vi "Psych Chart Look-up BY RH.vi"(0 "Relative Humidity [%]":dbl=72.0, 5 "Air Pressure [psia]":dbl=14.7, 7 "1st known value":dbl=55.0, 12 "1st Known Index":u16(ring) items=["DB", "WB", "RH", "HR", "Gr", "Vol", "h", "Dp"]) -> (8 "Output Array":dbl[](array[numeric]))   [LabVIEW 2020]
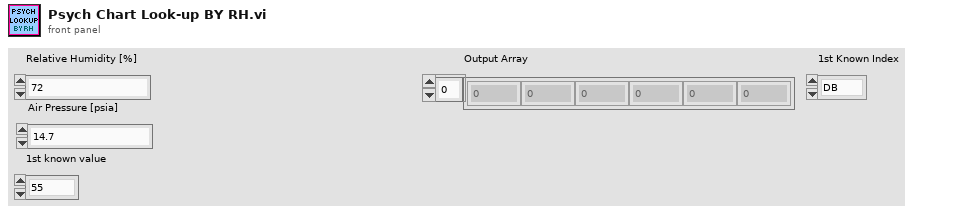
[diagram p1: front panel]
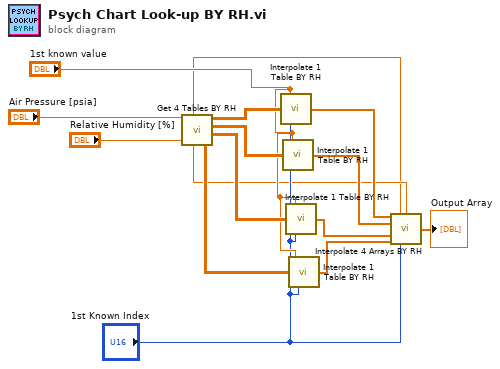
[diagram p0: block diagram]
diagram:
  n1 = call "Get 4 Tables BY RH.vi"("Air Pressure [psia]"="Air Pressure [psia]", "Relative Humidity [%]"="Relative Humidity [%]") -> ("Pressure Z"=w2:dbl, "RH Z"=w3:dbl, "HP Higher RH Psych Table"=w13:dbl[][], "HP Lower RH Psych Table"=w12:dbl[][], "LP Higher RH Psych Table"=w11:dbl[][], "LP Lower RH Psych Table"=w10:dbl[][])  [unwired: 1 in]
  n2 = call "Interpolate 1 Table BY RH.vi"("First Known Value"="1st known value", "Psych Table, 1 Press., 1 RH"=w13, "First Known Index"="1st Known Index") -> ("Output Array"=w9:dbl[])  [unwired: 12 in]
  n3 = call "Interpolate 1 Table BY RH.vi"("First Known Value"="1st known value", "Psych Table, 1 Press., 1 RH"=w12, "First Known Index"="1st Known Index") -> ("Output Array"=w8:dbl[])  [unwired: 12 in]
  n4 = call "Interpolate 1 Table BY RH.vi"("First Known Value"="1st known value", "Psych Table, 1 Press., 1 RH"=w11, "First Known Index"="1st Known Index") -> ("Output Array"=w7:dbl[])  [unwired: 12 in]
  n5 = call "Interpolate 1 Table BY RH.vi"("First Known Value"="1st known value", "Psych Table, 1 Press., 1 RH"=w10, "First Known Index"="1st Known Index") -> ("Output Array"=w6:dbl[])  [unwired: 12 in]
  n6 = call "Interpolate 4 Arrays BY RH.vi"("HP Higher RH Array"=w9, "Pressure Z"=w2, "RH Z"=w3, "HP Lower RH Array"=w8, "LP Higher RH Array"=w7, "LP Lower RH Array"=w6, "1st Known Index"="1st Known Index") -> ("Output Array"=→"Output Array":dbl[])  [unwired: 8 in]
